vi "ApproxRMS.vi"(8 "Reset":bool, 11 "Input":dbl) -> (3 "Approx RMS":dbl)   [LabVIEW 2010, in "KevLib01.lvlib"]
uses:
  KevLib01.lvlib
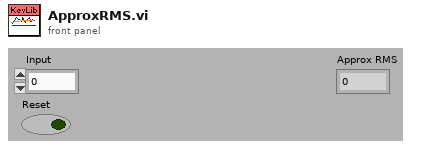
[diagram p1: front panel]
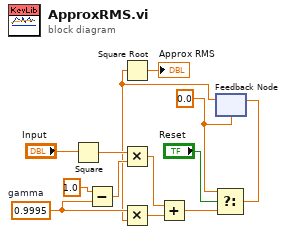
[diagram p0: block diagram]
diagram:
  w2 = 0.0 ("x")
  w8 = 0.9995  # gamma
  n1 = Square(x="Input") -> (x^2=w11:dbl)
  n2 = Subtract(x=1.0, y=w8) -> (x-y=w9:dbl)
  n3 = Multiply(x=w11, y=w9) -> (x*y=w7:dbl)
  n4 = feedback #1(w2) -> (w5:dbl)
  n5 = Square Root(x=w5) -> (sqrt(x)=→"Approx RMS":dbl)
  n6 = Multiply(x=w8, y=w5) -> (x*y=w6:dbl)
  n7 = Add(x=w7, y=w6) -> (x+y=w4:dbl)
  n8 = Select(t=w2, s="Reset", f=w4) -> (s? t:f=w3:dbl)
  n9 = feedback-in #1(w3) -> ()
